vi "AlliGator Is IRF Valid.vi"(2 "Reference Decay":cluster{"t Array":dbl[], "I Array":dbl[]}) -> (7 "Valid Plot?":bool)   [LabVIEW 2021, in "AlliGator Decay Analysis.lvlib" / "AlliGator Decay Fit.lvlib"]
doc: "Checks that the <B>Reference Decay</B> is a valid plot."
uses:
  AlliGator Decay Fit.lvlib
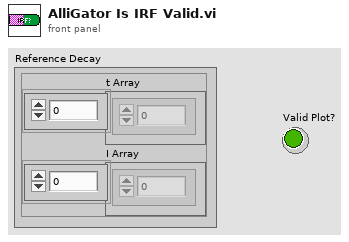
[diagram p1: front panel]
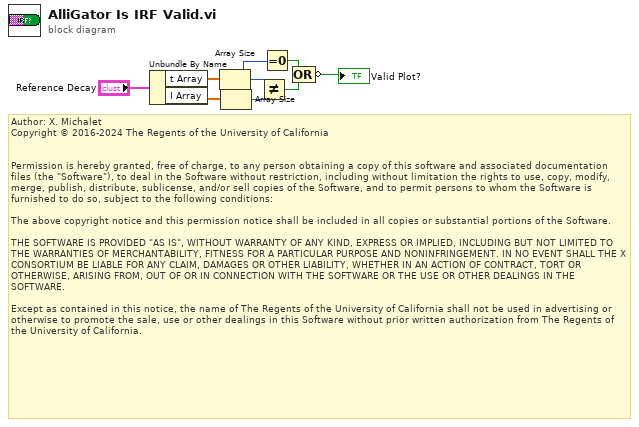
[diagram p0: block diagram]
diagram:
  # "Author: X. Michalet\nCopyright © 2016-2024 The Regents of the University of California\n \n\nPermission is hereby granted, free of charge, to any person obtaining a copy of this software and associated documentation files (the \"Software\"), to deal in the Software without restriction, including without limitation the rights to use, copy, modify, merge, publish, distribute, sublicense, and/or sell copies of the Software, and to permit persons to whom the Software is furnished to do so, subject to the following conditions:\n\nThe above copyright notice and this permission notice shall be included in all copies or substantial portions of the Software.\n\nTHE SOFTWARE IS PROVIDED \"AS IS\", WITHOUT WARRANTY OF ANY KIND, EXPRESS OR IMPLIED, INCLUDING BUT NOT LIMITED TO THE WARRANTIES OF MERCHANTABILITY, FITNESS FOR A PARTICULAR PURPOSE AND NONINFRINGEMENT. IN NO EVENT SHALL THE X CONSORTIUM BE LIABLE FOR ANY CLAIM, DAMAGES OR OTHER LIABILITY, WHETHER IN AN ACTION OF CONTRACT, TORT OR OTHERWISE, ARISING FROM, OUT OF OR IN CONNECTION WITH THE SOFTWARE OR THE USE OR OTHER DEALINGS IN THE SOFTWARE.\n\nExcept as contained in this notice, the name of The Regents of the University of California shall not be used in advertising or otherwise to promote the sale, use or other dealings in this Software without prior written authorization from The Regents of the University of California."
  n1 = Unbundle By Name("Reference Decay") -> ("t Array"=w7:dbl[], "I Array"=w6:dbl[])
  n2 = Array Size(array=w7) -> (size(s)=w4:i32)
  n3 = Array Size(array=w6) -> (size(s)=w5:i32)
  n4 = Not Equal?(x=w4, y=w5) -> (x != y?=w2:bool)
  n5 = Equal To 0?(x=w4) -> (x = 0?=w3:bool)
  n6 = Compound Arithmetic op=OR(w3, w2) -> (invert →"Valid Plot?":bool)
